vi "Inverse Time Curves (IEC, Dependent Reset).vi"(6 "operate time compensation":cluster{"G/Gs":dbl, "compensation [s]":dbl}[](array[cluster]), 7 "GD (25)":u16=25, 8 "error in (no error)":errorcluster, 9 "reset time parameters":T1={"tr [s]"=1.0, "alpha"=1.0}, 10 "time multiplier setting (1)":dbl=1.0, 11 "curve type":u16(ring) items=["IEC inverse", "IEC very inverse", "IEC extremely inverse"]) -> (0 "error out":errorcluster, 2 "memory size":u16, 3 "memory initial values":fxp<+,51,51>[](array[numeric]), 4 "curve data":cluster{"G/Gs":dbl[], "times [s]":dbl[]})   [LabVIEW 2014, in "NI_EP_Protection.lvlib"]
doc: "Generates memory initial values and memory size, which contain the information of the inverse time curves, for the FPGA Inverse Time Delay VI to use. You can compensate for the processing delay of the input energizing quantity under a specific G/Gs to achieve higher operate time accuracy."
uses:
  <vilib>/addons/Electrical Power/Protection/NI_EP_Protection.lvlib
  <vilib>/addons/Electrical Power/Protection/Inverse Time Delay/subVIs/ep_Reset Time.ctl
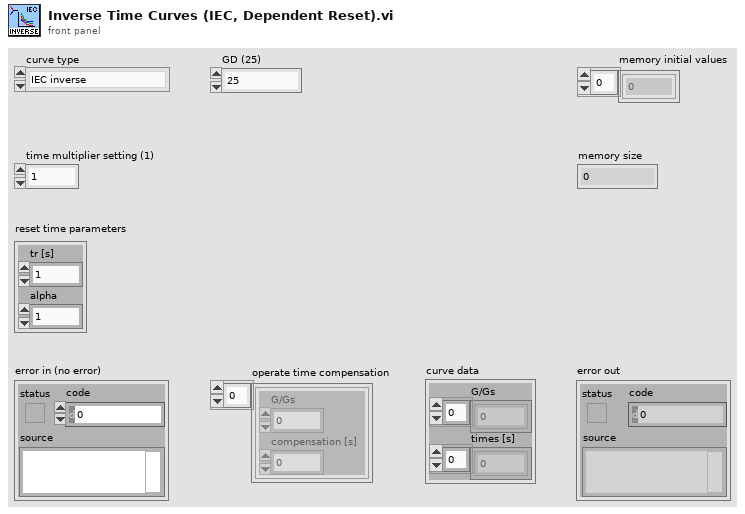
[diagram p1: front panel]
types:
  T1 = typedef "NI_EP_Protection.lvlib/ep_Reset Time.ctl" = cluster{"tr [s]":dbl, "alpha":dbl}
  T2 = typedef "NI_EP_Protection.lvlib/ep_Curve Parameters.ctl" = cluster{"operate time parameters":T3, "reset time parameters":T1}
  T3 = typedef "NI_EP_Protection.lvlib/ep_Operate Time.ctl" = cluster{"A [s]":dbl, "B [s]":dbl, "alpha":dbl, "K2 [s]":dbl, "K1 [s]":dbl, "K3 [s]":dbl}
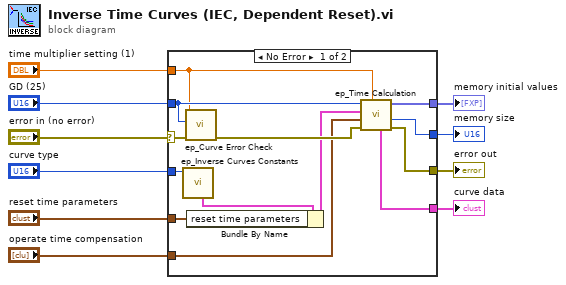
[diagram p0: block diagram]
diagram:
  n1 = case shown="No Error" "error in (no error)" {
    selector: "error in (no error)" -> [w21 w24]
    tunnel: [w16 w24] -> w9
    tunnel: "curve type" -> [w18 _]
    tunnel: [w17 _] -> w7
    tunnel: "reset time parameters" -> [w12 _]
    tunnel: "GD (25)" -> [w23 _]
    tunnel: "time multiplier setting (1)" -> [w22 _]
    tunnel: [w19 _] -> w3
    tunnel: [w15 _] -> w2
    tunnel: "operate time compensation" -> [w11 _]
    frame No Error {
      n2 = call <vilib>:"ep_Inverse Curves Constants.vi"("IEC curve type"=w18) -> ("IEC parameters"=w14:T2)  [unwired: 5 in, 5 out]
      n3 = call <vilib>:"ep_Curve Error Check.vi"("error in (no error)"=w21, "GD"=w23, "time dial"=w22) -> ("error out"=w20:errorcluster)  [unwired: 8 in]
      n4 = Bundle By Name(cluster=w14, "reset time parameters"=w12) -> (w13:T2)
      n5 = call <vilib>:"ep_Time Calculation.vi"("time dial"=w22, "error in (no error)"=w20, "operate time compensation"=w11, "curve parameters"=w13, "GD"=w23) -> ("error out"=w16:errorcluster, "memory size"=w19:u16, "memory initial values"=w17:fxp<+,51,51>[], "curve data"=w15:cluster{"G/Gs":dbl[], "times":dbl[]})  [unwired: 3 in]
    }
    frame Error {
    }
  }
  "memory initial values" <- w7
  "error out" <- w9
  "memory size" <- w3
  "curve data" <- w2
